vi "test_Lunit_Verify.vi"(8 "error in (no error)":errorcluster, 11 "My Test Case Lunit in":refnum<class "My Test Case Lunit.lvclass">) -> (0 "error out":errorcluster, 3 "My Test Case Lunit out":refnum<class "My Test Case Lunit.lvclass">)   [LabVIEW 2020, in "My Test Case Lunit.lvclass"]
uses:
  My Test Case Lunit.lvclass
  My Test Case Lunit.lvclass/My Test Case Lunit.ctl
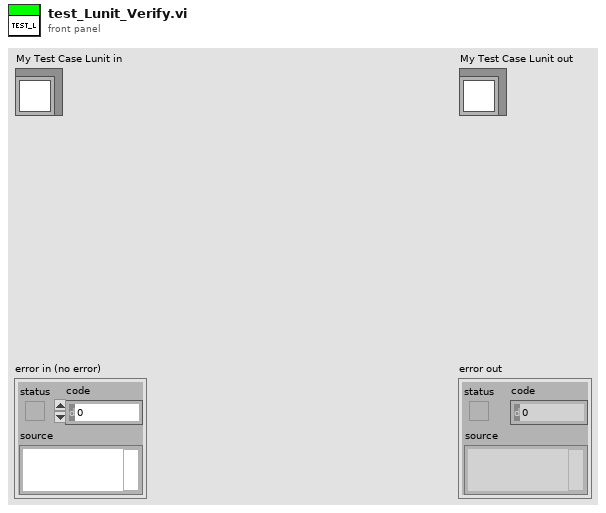
[diagram p1: front panel]
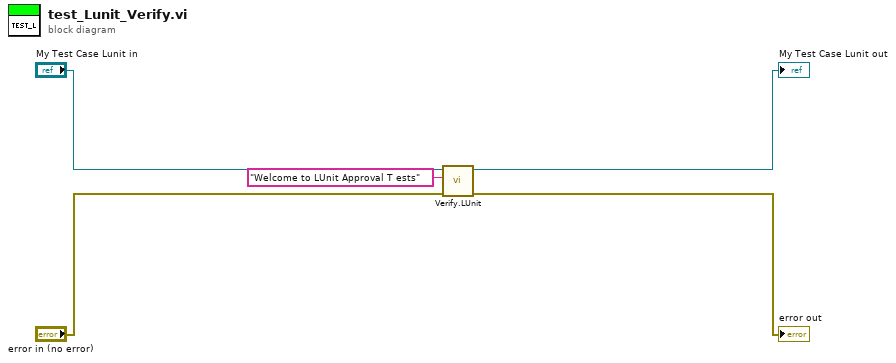
[diagram p0: block diagram]
diagram:
  n1 = call "Verify.LUnit.vi"("error in (no error)"="error in (no error)", "Test Data"="Welcome to LUnit Approval T ests", "My Test Case Lunit in"="My Test Case Lunit in") -> ("error out"=→"error out":errorcluster, "My Test Case Lunit out"=→"My Test Case Lunit out":refnum<class "My Test Case Lunit.lvclass">)  [unwired: 7 in]
